vi "Nachtmessung_Moden.vi"() -> ()   [LabVIEW 2010]
panel:
  in  "error in (no error)":errorcluster
  out "error out":errorcluster
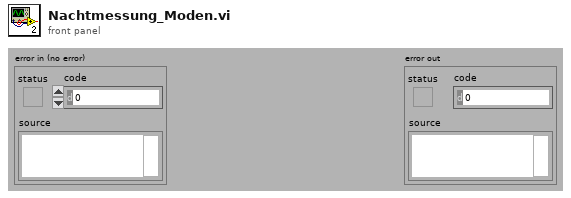
[diagram p1: front panel]
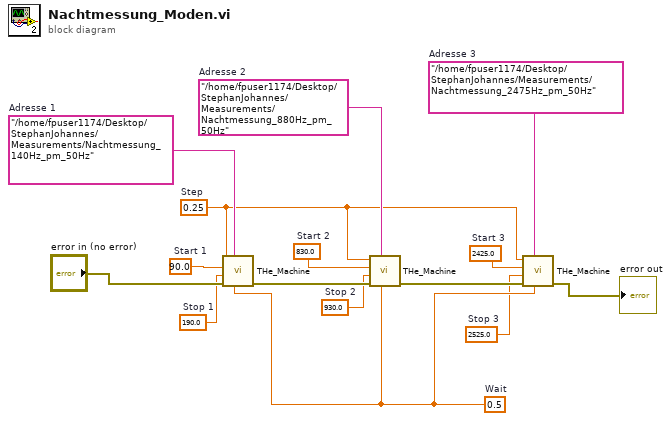
[diagram p0: block diagram]
diagram:
  w3 = "/home/fpuser1174/Desktop/StephanJohannes/Measurements/Nachtmessung_2475Hz_pm_50Hz"  # Adresse 3
  w4 = "/home/fpuser1174/Desktop/StephanJohannes/Measurements/Nachtmessung_880Hz_pm_50Hz"  # Adresse 2
  w2 = "/home/fpuser1174/Desktop/StephanJohannes/Measurements/Nachtmessung_140Hz_pm_50Hz"  # Adresse 1
  w6 = 2525.0  # Stop 3
  w5 = 2425.0  # Start 3
  w8 = 930.0  # Stop 2
  w9 = 830.0  # Start 2
  w1 = 0.25  # Step
  w13 = 190.0  # Stop 1
  w14 = 90.0  # Start 1
  w7 = 0.5  # Wait
  n1 = call "THe_Machine.vi"("Wait"=w7, "Adresse"=w2, "error in (no error)"="error in (no error)", "Stop Frequency"=w13, "Start Frequency"=w14, "Stepsize"=w1) -> ("error out"=w12:errorcluster)  [unwired: 4 out]
  n2 = call "THe_Machine.vi"("Wait"=w7, "Adresse"=w4, "error in (no error)"=w12, "Stop Frequency"=w8, "Start Frequency"=w9, "Stepsize"=w1) -> ("error out"=w11:errorcluster)  [unwired: 4 out]
  n3 = call "THe_Machine.vi"("Wait"=w7, "Adresse"=w3, "error in (no error)"=w11, "Stop Frequency"=w6, "Start Frequency"=w5, "Stepsize"=w1) -> ("error out"=→"error out":errorcluster)  [unwired: 4 out]
